vi "Execute.vi"(8 "error in (no error)":errorcluster, 10 "ObserverRegistry in":refnum<class "ObserverRegistry.lvclass">, 11 "ObserverRegistryCommand":refnum<class "Observer_RegisterForAll.lvclass">) -> (0 "error out":errorcluster, 2 "ObserverRegistry out":refnum<class "ObserverRegistry.lvclass">, 3 "Message":refnum<class "MSG.lvclass">)   [LabVIEW 2011, in "Messenging.lvlib" / "Observer_RegisterForAll.lvclass"]
uses:
  Observer_RegisterForAll.lvclass
  ObserverRegistry.lvclass
  ParentCommand/ObserverRegistryCommand.lvclass
  Messenging.lvlib
  Interprocess Messenger/TextVarientMessage/MSG.lvclass
  Registration Entry.ctl
  Interprocess Messenger/SendMultiple/Create Observer.vi
  Interprocess Messenger/SendMultiple/ObserverSet.lvclass
  Interprocess Messenger/Send/Send.lvclass
  Interprocess Messenger/SendOnly/Observer.lvclass
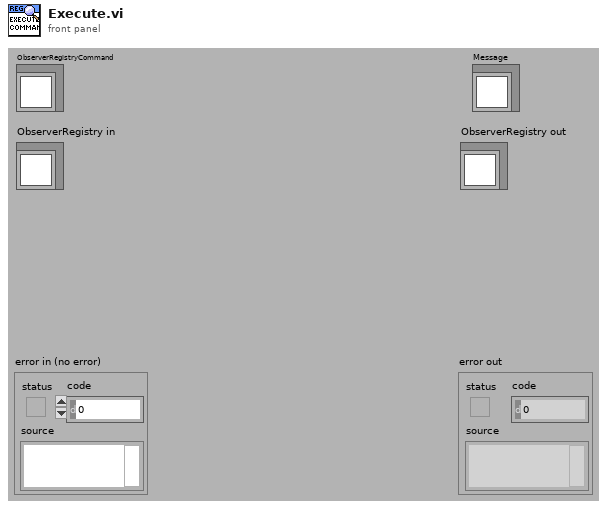
[diagram p1: front panel]
types:
  T1 = typedef "Messenging.lvlib/ObserverRegistry.lvclass/ObserverRegistryData.ctl" = cluster{"Observer of Errors":refnum<class "Observer.lvclass">, "Observer of All":refnum<class "Observer.lvclass">, "Event Registry":variant}
  T2 = typedef "Messenging.lvlib/ObserverRegistry.lvclass/Registration Entry.ctl" = cluster{"Observer":refnum<class "Observer.lvclass">, "Type":enum16{"Event", "State"}, "Latest (State)":refnum<class "MSG.lvclass">}
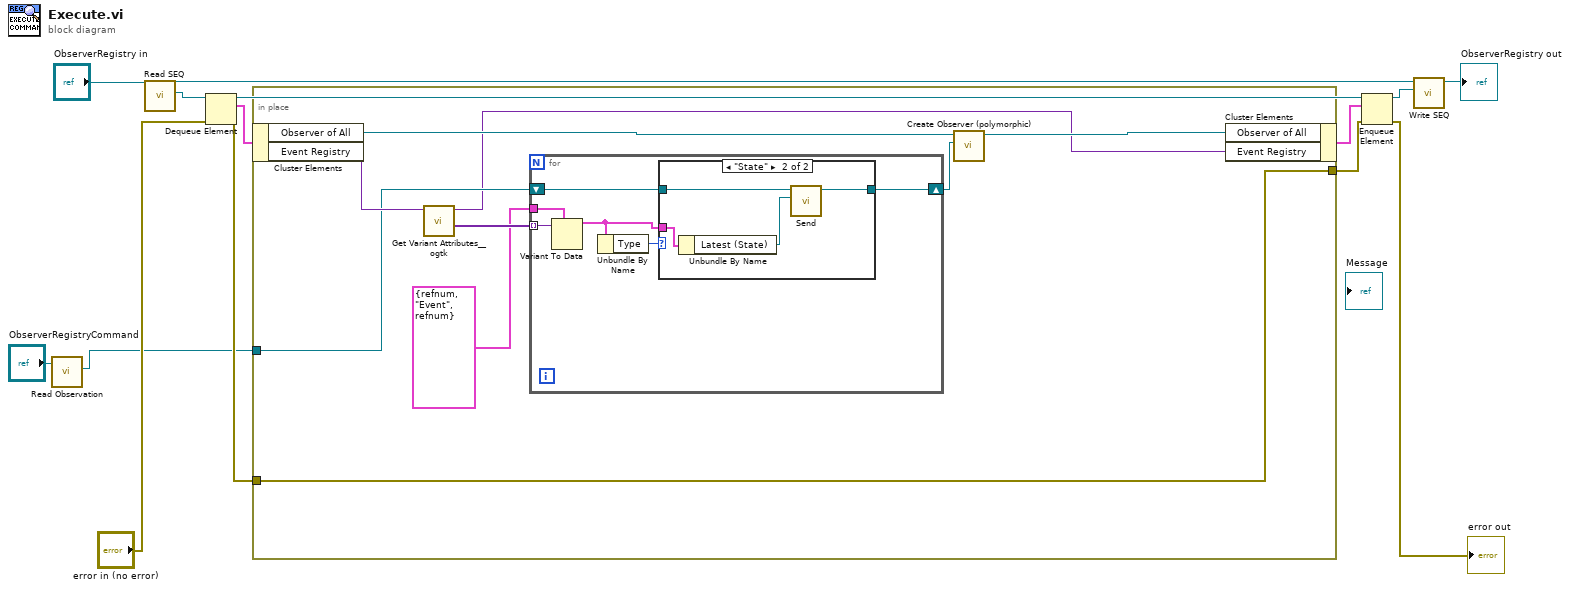
[diagram p0: block diagram]
diagram:
  n1 = call "Read Observation.vi"("ObserverRegistryCommand.lvclass in"="ObserverRegistryCommand") -> ("Observer"=w1:refnum<class "Send.lvclass">)  [unwired: 1 in, 9 out]
  n2 = call "Read SEQ.vi"("ObserverRegistry.lvclass in"="ObserverRegistry in") -> ("SEQ"=w7:refnum<queue>, "ObserverRegistry.lvclass out"=w5:refnum<class "ObserverRegistry.lvclass">)  [unwired: 1 in, 8 out]
  n3 = Dequeue Element(queue=w7, error in (no error)="error in (no error)") -> (queue out=w12:refnum<queue>, element=w14:T1, error out=w10:errorcluster)  [unwired: 2 out]
  n4 = in-place {
    in-place-border: w10 -> [w21]
    in-place-border: w1 -> [w17]
    in-place-border: [w21] -> w2
    n5 = in-place-cluster #1(w14) -> ("Observer of All"=w23:refnum<class "Observer.lvclass">, "Event Registry"=w20:variant)
    n6 = call <userlib>:"Get Variant Attributes__ogtk.vi"("Variant"=w20) -> ("value(s)"=w19:variant[], "duplicate Variant"=w15:variant)  [unwired: 1 in, 4 out]
    n7 = for {
      tunnel: w19 -> [w29] mode=indexing
      tunnel: T2 {"Observer"=refnum, "Type"=enum."Event", "Latest (State)"=refnum} ("Registration Entry") -> [w28]
      shift-right: [w24] -> w16
      shift-left: w17 -> [w25]
      n8 = Variant To Data(type=w28, Variant=w29) -> (data=w26:T2)  [unwired: 1 in, 1 out]
      n9 = Unbundle By Name(w26) -> ("Type"=w27:enum16{"Event", "State"})
      n10 = case shown="\"State\"" w27 {
        tunnel: w26 -> [_ w34]
        tunnel: w25 -> [w30 w33]
        tunnel: [w30 w31] -> w24
        frame "Event", Default {
        }
        frame "State" {
          n11 = Unbundle By Name(w34) -> ("Latest (State)"=w32:refnum<class "MSG.lvclass">)
          n12 = call-dynamic "Send.vi"("Message"=w32, "MSR Parent in"=w33) -> ("MSR Parent out"=w31:refnum<class "Send.lvclass">)  [unwired: 1 in, 8 out]
        }
      }
    }
    n13 = call-poly "Create Observer (polymorphic).vi"("Additional Input"=w16, "Input"=w23) -> ("Observer"=w22:refnum<class "Observer.lvclass">)  [unwired: 7 out]
    n14 = in-place-cluster #1("Observer of All"=w22, "Event Registry"=w15) -> (w13:T1)
  }
  n15 = Enqueue Element(queue=w12, element=w13, error in (no error)=w2) -> (queue out=w4:refnum<queue>, error out=→"error out":errorcluster)  [unwired: 2 out]
  n16 = call "Write SEQ.vi"("SEQ"=w4, "ObserverRegistry.lvclass in"=w5) -> ("ObserverRegistry.lvclass out"=→"ObserverRegistry out":refnum<class "ObserverRegistry.lvclass">)  [unwired: 1 in, 8 out]
